vi "Helper SubVI - Padding Zeroes for Resample.vi"(4 "padding zeroes?":bool=TRUE, 9 "dt":dbl=1.0, 10 "delay":dbl, 11 "X":dbl[](array[numeric])) -> (2 "length of Y":i32, 3 "length of padding zeros":i32)   [LabVIEW 2023]
doc: "Determine the length of padding zeroes needed in order to get the resampled signal of the same time span as the input signal X."
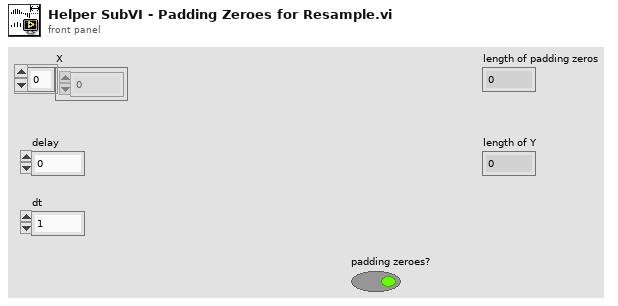
[diagram p1: front panel]
types:
  T1 = cluster{"new sample period":dbl, "Timing Jitter":enum32{"Interpolation", "Rounding"}, "first point location":dbl, "prototype filter":cluster{"h":dbl[], "Max Decimation":i32}}
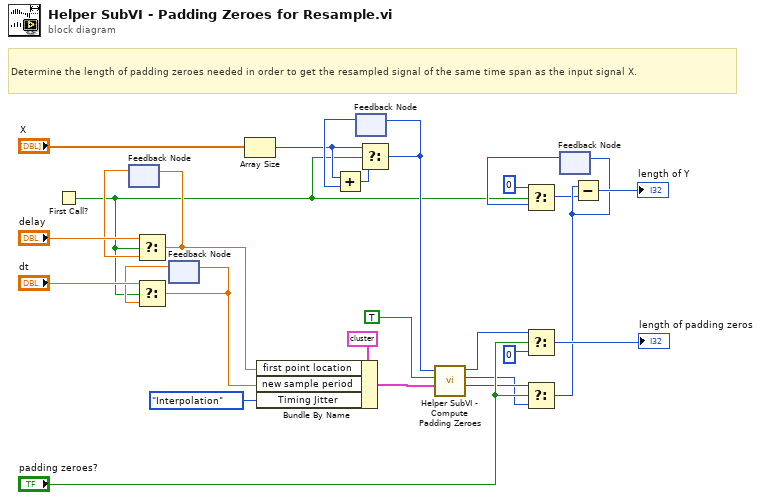
[diagram p0: block diagram]
diagram:
  # "Determine the length of padding zeroes needed in order to get the resampled signal of the same time span as the input signal X."
  n1 = First Call?() -> (First Call?: T/F=w2:bool)
  n2 = feedback #1() -> (w16:dbl)  [unwired: 1 in]
  n3 = Select(t="delay", s=w2, f=w16) -> (s? t:f=w17:dbl)
  n4 = feedback-in #1(w17) -> ()
  n5 = feedback #2() -> (w14:dbl)  [unwired: 1 in]
  n6 = Select(t="dt", s=w2, f=w14) -> (s? t:f=w15:dbl)
  n7 = feedback-in #2(w15) -> ()
  n8 = Array Size(array="X") -> (size(s)=w10:i32)
  n9 = Bundle By Name(cluster=T1 {"new sample period"=0.0, "Timing Jitter"=enum."Interpolation", "first point location"=0.0, "prototype filter"={"h"=array[10231 elements], "Max Decimation"=128}} ("config"), "first point location"=w17, "new sample period"=w15, "Timing Jitter"=enum32{"Interpolation", "Rounding"}."Interpolation" ("timing jitter")) -> (w9:T1)
  n10 = feedback #3() -> (w20:i32)  [unwired: 1 in]
  n11 = Add(x=w10, y=w20) -> (x+y=w11:i32)
  n12 = Select(t=w10, s=w2, f=w11) -> (s? t:f=w21:i32)
  n13 = feedback-in #3(w21) -> ()
  n14 = call "Helper SubVI - Compute Padding Zeroes.vi"("config"=w9, "anti-aliasing?"=TRUE, "length of X"=w21) -> ("length of Y (after padding zeroes)"=w4:i32, "length of Y"=w3:i32, "length of padding zeroes"=w8:i32)  [unwired: 6 in]
  n15 = Select(t=w8, s="padding zeroes?", f=0) -> (s? t:f=→"length of padding zeros":i32)
  n16 = Select(t=w4, s="padding zeroes?", f=w3) -> (s? t:f=w19:i32)
  n17 = feedback #4() -> (w18:i32)  [unwired: 1 in]
  n18 = Select(t=0, s=w2, f=w18) -> (s? t:f=w6:i32)
  n19 = feedback-in #4(w19) -> ()
  n20 = Subtract(x=w19, y=w6) -> (x-y=→"length of Y":i32)
